vi "GT_SetUserSegNum.vi"(8 "fifo":i16, 9 "SegNum":i32, 10 "crd":i16, 11 "rtn_In":cluster{"rtn":i16, "Func":string}) -> (1 "fifo out":i16, 2 "crd out":i16, 3 "rtn_Out":cluster{"rtn":i16, "Func":string})   [LabVIEW 2014]
uses:
  VC6/gts.dll
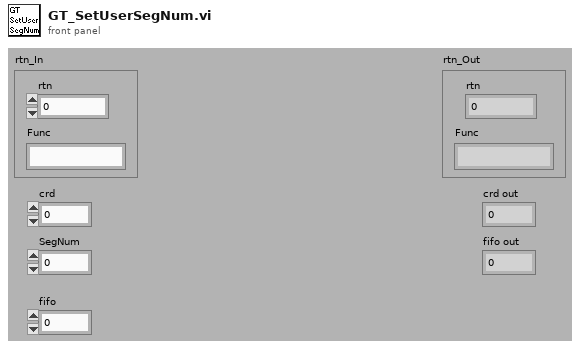
[diagram p1: front panel]
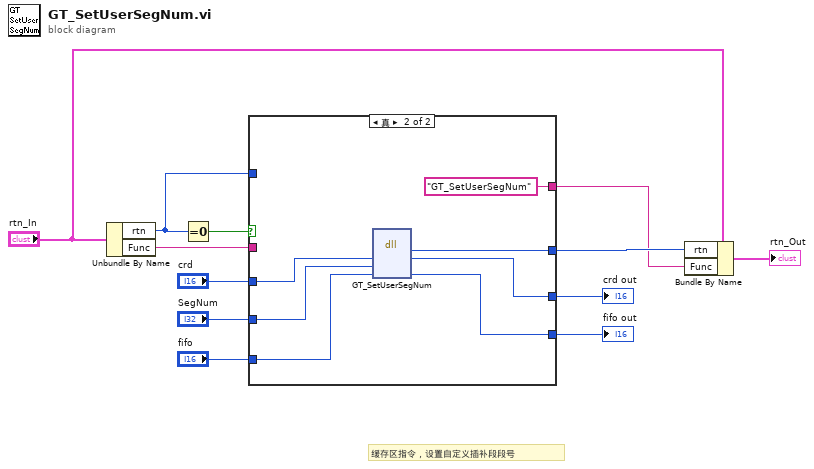
[diagram p0: block diagram]
diagram:
  # "缓存区指令，设置自定义插补段段号"
  n1 = Unbundle By Name("rtn_In") -> ("rtn"=w2:i16, "Func"=w1:string)
  n2 = Equal To 0?(x=w2) -> (x = 0?=w12:bool)
  n3 = case shown="真" w12 {
    tunnel: [w16 w23] -> w9
    tunnel: [w15 "GT_SetUserSegNum" ("Func")] -> w8
    tunnel: "crd" -> [w14 w21]
    tunnel: "SegNum" -> [_ w20]
    tunnel: "fifo" -> [w13 w19]
    tunnel: [w14 w18] -> w4
    tunnel: [w13 w17] -> w3
    tunnel: w2 -> [w16 _]
    tunnel: w1 -> [w15 _]
    frame False {
    }
    frame True {
      n4 = dll-call lib="PTH2Fabs DNewGTS AC-800LWin7版源程序-20170926gts85VC6gts.dll" fn="GT_SetUserSegNum"("crd"=w21, "SegNum"=w20, "fifo"=w19) -> ("rtn"=w23:i16, "crd"=w18:i16, "fifo"=w17:i16)  [unwired: 4 in, 2 out]
    }
  }
  "crd out" <- w4
  "fifo out" <- w3
  n5 = Bundle By Name(cluster="rtn_In", "rtn"=w9, "Func"=w8) -> (→"rtn_Out":cluster{"rtn":i16, "Func":string})
